vi "Supply_SetVolts.vi"(8 "error in (no error)":errorcluster, 9 "Command string":string, 10 "Volts IN [V]":dbl, 11 "KE2410 in":refnum<class "KE2410.lvclass">) -> (0 "error out":errorcluster, 2 "Compliance exceeded?":bool, 3 "KE2410 out":refnum<class "KE2410.lvclass">)   [LabVIEW 2013, in "KE2410.lvclass"]
uses:
  KE2410.lvclass
  SupplyControl.lvclass
  InstrumentSetup.vi
  InstrControl.lvclass
panel:
  out "Command sent":string
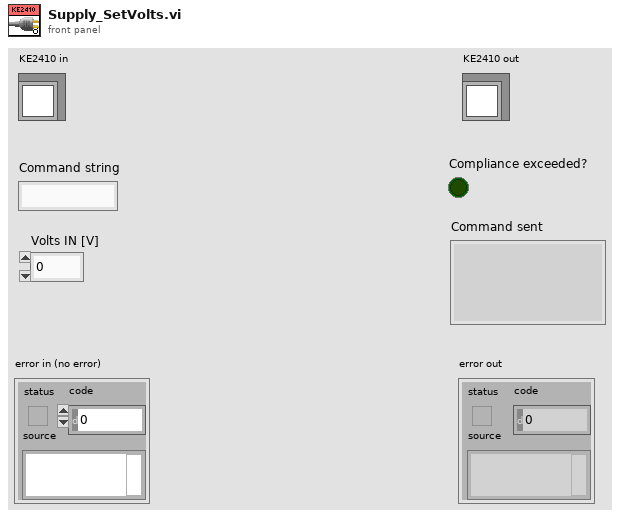
[diagram p1: front panel]
types:
  T1 = cluster{"Current Limit":sgl, "Front/Rear Output:":u16, "KE2410":refnum<class "KE2410.lvclass">}
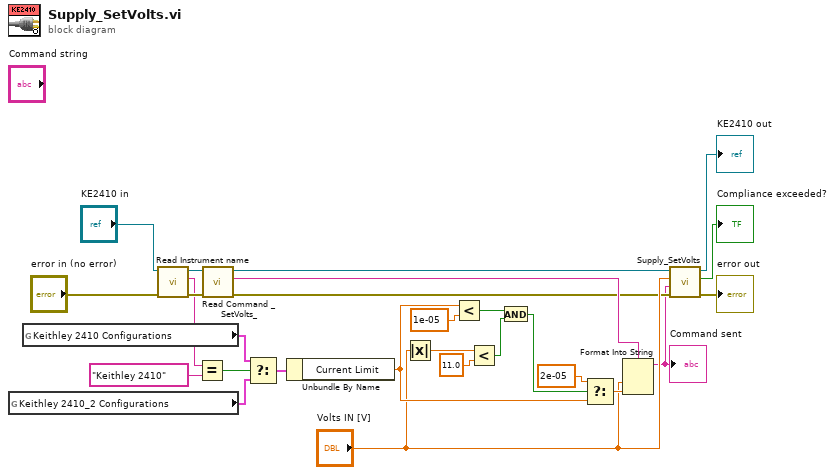
[diagram p0: block diagram]
diagram:
  n1 = global read "InstrumentSetup.vi" "Keithley 2410_2 Configurations"() -> (w2:T1)
  n2 = global read "InstrumentSetup.vi" "Keithley 2410 Configurations"() -> (w3:T1)
  n3 = call-dynamic "Read Instrument name.vi"("error in (no error)"="error in (no error)", "InstControl in"="KE2410 in") -> ("error out"=w9:errorcluster, "Instrument name"=w5:string, "InstControl out"=w7:refnum<class "KE2410.lvclass">)  [unwired: 7 in]
  n4 = Equal?(x=w5, y="Keithley 2410") -> (x = y?=w4:bool)
  n5 = call-dynamic "Read Command _SetVolts_.vi"("error in (no error)"=w9, "SupplyControl in"=w7) -> ("error out"=w13:errorcluster, "Command \"SetVolts\""=w14:string, "SupplyControl out"=w12:refnum<class "KE2410.lvclass">)  [unwired: 7 in]
  n6 = Select(t=w3, s=w4, f=w2) -> (s? t:f=w1:T1)
  n7 = Unbundle By Name(w1) -> ("Current Limit"=w16:sgl)
  n8 = Absolute Value(x="Volts IN [V]") -> (abs(x)=w17:dbl)
  n9 = Less?(x=w16, y=1e-05) -> (x < y?=w21:bool)
  n10 = Less?(x=w17, y=11.0) -> (x < y?=w19:bool)
  n11 = And(x=w21, y=w19) -> (x .and. y?=w20:bool)
  n12 = Select(t=2e-05, s=w20, f=w16) -> (s? t:f=w24:dbl)
  n13 = Format Into String(format string=w14, "Volts IN [V]", w24) -> (resulting string=w11:string)  [unwired: 2 in, 1 out]
  "Command sent" <- w11
  n14 = call-parent "Supply_SetVolts.vi"("error in (no error)"=w13, "Command string"=w11, "Volts IN [V]"="Volts IN [V]", "SupplyControl in"=w12) -> ("error out"=→"error out":errorcluster, "Compliance exceeded?"=→"Compliance exceeded?":bool, "SupplyControl out"=→"KE2410 out":refnum<class "KE2410.lvclass">)  [unwired: 5 in]
